vi "Normalised values precision.vi"() -> (3 "Normalised values precision":i32)   [LabVIEW 2017]
panel:
  # "SUBROUTINE"
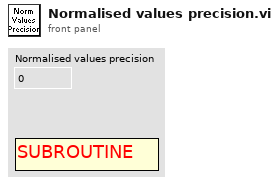
[diagram p1: front panel]
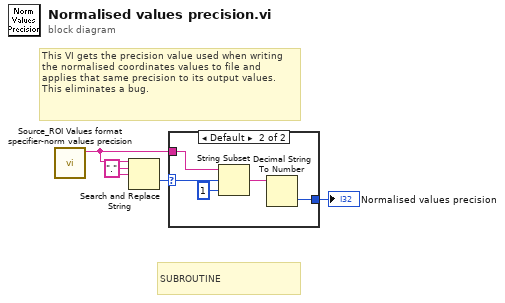
[diagram p0: block diagram]
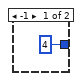
[diagram p2: hidden frame]
diagram:
  w1 = "." ("search string")
  # "SUBROUTINE"
  # "This VI gets the precision value used when writing the normalised coordinates values to file and applies that same precision to its output values. This eliminates a bug."
  n1 = call "Source_ROI Values format specifier-norm values precision.vi"() -> ("format (%.3f)"=w3:string)  [unwired: 11 in]
  n2 = Search and Replace String(input string=w3, search string=w1, replace string=w1) -> (offset past replacement=w2:i32)  [unwired: 5 in, 3 out]
  n3 = case shown="Default" w2 {
    selector: w2 -> [_ w9]
    tunnel: w3 -> [_ w8]
    tunnel: [4 w6] -> w4
    frame -1 {
    }
    frame Default {
      n4 = String Subset(string=w8, offset (0)=w9, length (rest)=1 ("length (rest)")) -> (substring=w7:string)
      n5 = Decimal String To Number(string=w7) -> (number=w6:i32)  [unwired: 2 in, 1 out]
    }
  }
  "Normalised values precision" <- w4
